vi "Append VI List of Controls to Report (refnum).vi"(0 "report in":refnum<class "NI_report.lvclass">, 1 "include only controls in con pane?":bool, 2 "image format (jpeg)":enum32{"PNG", "JPEG", "GIF"}(ring)=enum."JPEG", 5 "VI":refnum<vi>, 7 "alignment (default)":T2, 11 "error in (no error)":errorcluster, 12 "include control descriptions?":bool, 13 "include control data types?":bool, 14 "MS Office parameters":T1) -> (4 "report out":refnum<class "NI_report.lvclass">, 6 "VI out":refnum<vi>, 8 "start out (Word)":i32, 10 "end out (Word)":i32, 15 "error out":errorcluster)   [LabVIEW 2017, in "NI_ReportGenerationCore.lvlib"]
doc: "Appends a list of controls and indicators of the VI you specify in <B>VI</B> to a report. Wire data to the <B>VI</B> input to determine the polymorphic instance to use or manually select the instance."
uses:
  <vilib>/Utility/NIReport.llb/NI_ReportGenerationCore.lvlib
  <vilib>/Utility/NIReport.llb/NI_report.lvclass
  <vilib>/Utility/NIReport.llb/HTML Report Image Alignment.ctl
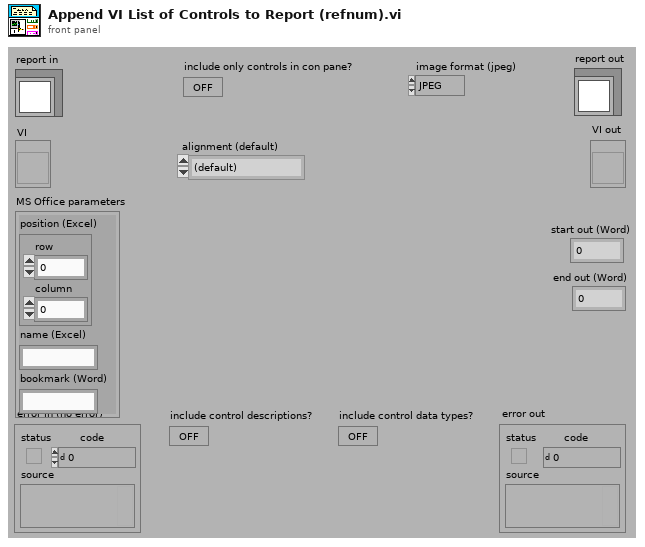
[diagram p1: front panel]
types:
  T1 = cluster{"position (Excel)":cluster{"row":i32, "column":i32}, "name (Excel)":string, "bookmark (Word)":string}
  T2 = typedef "NI_ReportGenerationCore.lvlib/HTML Report Image Alignment.ctl" = enum16{"(default)", "LEFT", "RIGHT", "TOP", "TEXTTOP", "MIDDLE", "ABSMIDDLE", "BASELINE", "BOTTOM", "ABSBOTTOM"}
  T3 = enum32{"invalid app kind", "Development System", "Run Time System", "Student Edition", "Embedded LabVIEW", "Evaluation", "Custom"}
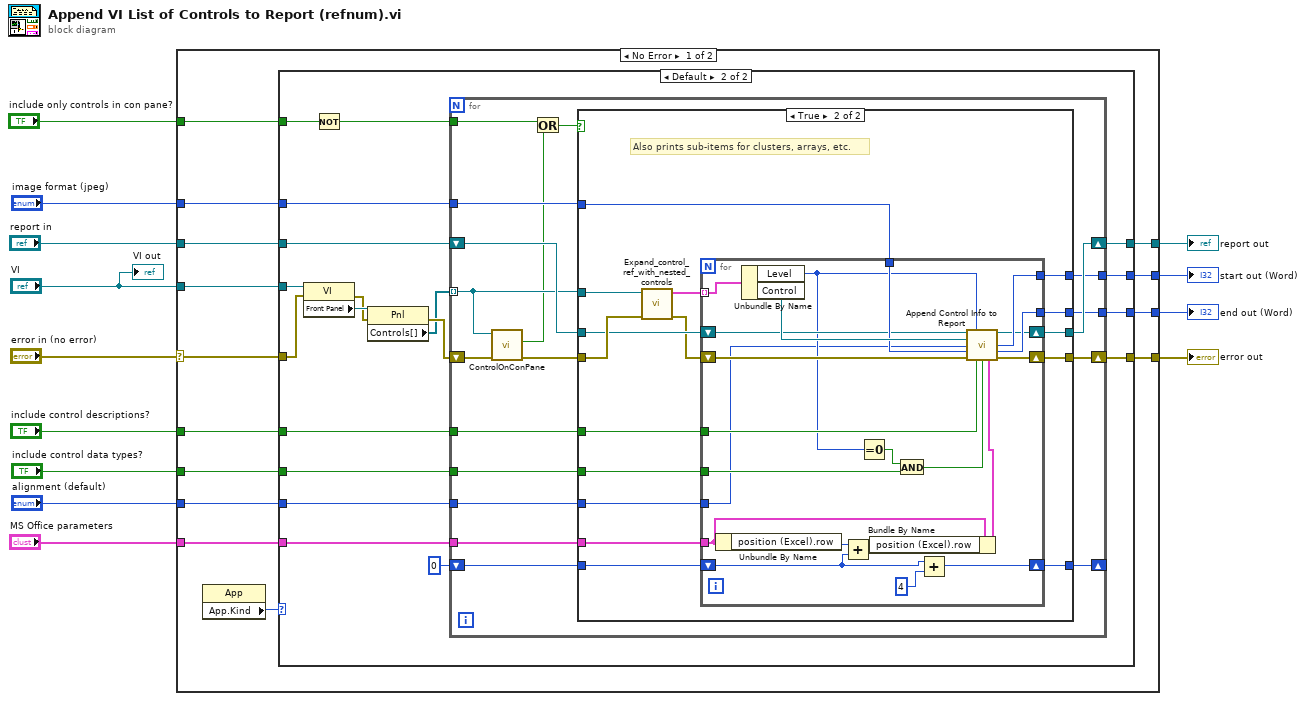
[diagram p0: block diagram]
diagram:
  n1 = case shown="No Error" "error in (no error)" {
    selector: "error in (no error)" -> [w21 w109]
    tunnel: [w26 w109] -> w12
    tunnel: "report in" -> [w24 w108]
    tunnel: "VI" -> [w22 _]
    tunnel: "image format (jpeg)" -> [w23 _]
    tunnel: "include control descriptions?" -> [w27 _]
    tunnel: "include control data types?" -> [w25 _]
    tunnel: "include only controls in con pane?" -> [w20 _]
    tunnel: "alignment (default)" -> [w19 _]
    tunnel: "MS Office parameters" -> [w18 _]
    tunnel: [w16 w108] -> w3
    tunnel: [w15 _] -> w2
    tunnel: [w14 _] -> w1
    frame No Error {
      n2 = property class="App"() -> ("App.Kind"=w17:T3)  [unwired: 2 in, 2 out]
      n3 = case shown="Default" w17 {
        tunnel: w27 -> [_ w48]
        tunnel: [w29 w47] -> w26
        tunnel: w25 -> [_ w46]
        tunnel: w24 -> [w28 w45]
        tunnel: w23 -> [_ w44]
        tunnel: w22 -> [_ w43]
        tunnel: w21 -> [w29 w40]
        tunnel: w20 -> [_ w38]
        tunnel: w19 -> [_ w36]
        tunnel: w18 -> [_ w33]
        tunnel: [w28 w32] -> w16
        tunnel: [_ w31] -> w15
        tunnel: [_ w30] -> w14
        frame "Run Time System" {
          # "Do not try to append\nif running in an\nexecutable"
        }
        frame Default {
          n4 = property class="VI"(reference=w43, error in=w40) -> (error out=w41:errorcluster, "Front Panel"=w42:refnum<vi>)  [unwired: 1 out]
          n5 = Not(x=w38) -> (.not. x?=w37:bool)
          n6 = property class="Pnl"(reference=w42, error in=w41) -> (error out=w39:errorcluster, "Controls[]"=w35:refnum<vi>[])  [unwired: 1 out]
          n7 = for {
            shift-right: [w65] -> w47
            shift-left: w39 -> [w58]
            tunnel: w48 -> [w66]
            tunnel: w46 -> [w64]
            tunnel: w44 -> [w62]
            tunnel: w35 -> [w59] mode=indexing
            tunnel: w37 -> [w61]
            tunnel: w36 -> [w55]
            shift-right: [w53] -> _
            shift-left: 0 -> [w54]
            tunnel: w33 -> [w52]
            shift-right: [w51] -> w32
            shift-left: w45 -> [w63]
            tunnel: [w50] -> w31
            tunnel: [w49] -> w30
            n8 = call <vilib>:"ControlOnConPane.vi"("error in (no error)"=w58, "Ctl Refnum"=w59) -> ("error out"=w57:errorcluster, "Is connected to connector pane?"=w56:bool)  [unwired: 7 in, 1 out]
            n9 = Or(x=w61, y=w56) -> (x .or. y?=w60:bool)
            n10 = case shown="True" w60 {
              tunnel: w66 -> [_ w78]
              tunnel: [w69 w80] -> w65
              tunnel: w64 -> [_ w77]
              tunnel: w57 -> [w69 w85]
              tunnel: w63 -> [w67 w84]
              tunnel: w62 -> [_ w79]
              tunnel: w59 -> [_ w83]
              tunnel: w55 -> [_ w76]
              tunnel: w52 -> [_ w75]
              tunnel: w54 -> [w68 w74]
              tunnel: [w68 w73] -> w53
              tunnel: [w67 w72] -> w51
              tunnel: [_ w71] -> w50
              tunnel: [_ w70] -> w49
              frame False {
              }
              frame True {
                # "Also prints sub-items for clusters, arrays, etc."
                n11 = call <vilib>:"Expand_control_ref_with_nested_controls.vi"("error in (no error)"=w85, "Control"=w83) -> ("error out"=w81:errorcluster, "Array of control info"=w82:cluster{"Control":refnum<vi>, "Level":i32}[])  [unwired: 4 in]
                n12 = for {
                  tunnel: w82 -> [w107] mode=indexing
                  shift-right: [w105] -> w80
                  shift-left: w81 -> [w101]
                  tunnel: w79 -> [w104]
                  tunnel: w78 -> [w102]
                  tunnel: w77 -> [w98]
                  tunnel: w76 -> [w96]
                  tunnel: [w95] -> w70
                  tunnel: [w94] -> w71
                  tunnel: w75 -> [w90]
                  shift-right: [w87] -> w73
                  shift-left: w74 -> [w89]
                  shift-right: [w86] -> w72
                  shift-left: w84 -> [w103]
                  n13 = Unbundle By Name(w90) -> ("position (Excel).row"=w93:i32)
                  n14 = Unbundle By Name(w107) -> ("Level"=w100:i32, "Control"=w106:refnum<vi>)
                  n15 = Add(x=w93, y=w89) -> (x+y=w92:i32)
                  n16 = Equal To 0?(x=w100) -> (x = 0?=w99:bool)
                  n17 = Bundle By Name(cluster=w90, "position (Excel).row"=w92) -> (w91:T1)
                  n18 = And(x=w99, y=w98) -> (x .and. y?=w97:bool)
                  n19 = Add(x=w89, y=4) -> (x+y=w87:i32)
                  n20 = call <vilib>:"Append Control Info to Report.vi"("report in"=w103, "level"=w100, "ctl refnum"=w106, "alignment (default)"=w96, "image format (jpeg)"=w104, "error in"=w101, "include control descriptions?"=w102, "include control datatype information?"=w97, "MS Office parameters"=w91) -> ("report out"=w86:refnum<class "NI_report.lvclass">, "start out (word)"=w95:i32, "end out (word)"=w94:i32, "error out"=w105:errorcluster)  [unwired: 3 in]
                }
              }
            }
          }
        }
      }
    }
    frame Error {
    }
  }
  "error out" <- w12
  "report out" <- w3
  "end out (Word)" <- w2
  "start out (Word)" <- w1
  "VI out" <- "VI"
